vi "VI Server_Get Text Ring Selection.vi"(7 "Label":string, 8 "error in":errorcluster, 9 "Single Instance (T)":bool=TRUE, 11 "VI Server Cluster":T1) -> (0 "error out":errorcluster, 1 "Control Reference":refnum<vi>, 2 "Selection":string, 3 "VI Server Custer.DUP":T1={"Labels"=["Label", "Size", "Font", "Heght", "Width", "Ledding Denominator", "Ledding Nominator", "Label Number", "Microstep Resolution", "X", "Y", "Z", "Italic?", "Underlined?"], "Refs"=[], "VI Ref"=refnum}, 4 "Value":u16, 6 "Label.Text":string)   [LabVIEW 2020, in "VI Server Toolkit LV2013.lvlib"]
doc: "Returns Item Name selected of the Text Ring."
uses:
  VI Server Toolkit LV2013.lvlib
  VI Server_TypeDefs/VI Server_RefsCluster.ctl
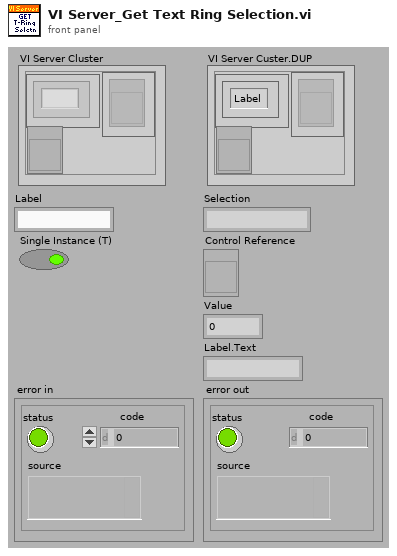
[diagram p1: front panel]
types:
  T1 = typedef "VI Server_RefsCluster.ctl" = cluster{"Labels":string[], "Refs":refnum<vi>[], "VI Ref":refnum<vi>}
  T2 = typedef "LVStringsAndValuesArrayTypeDef_U16.ctl" = cluster{"String":string, "Value":u16}[]
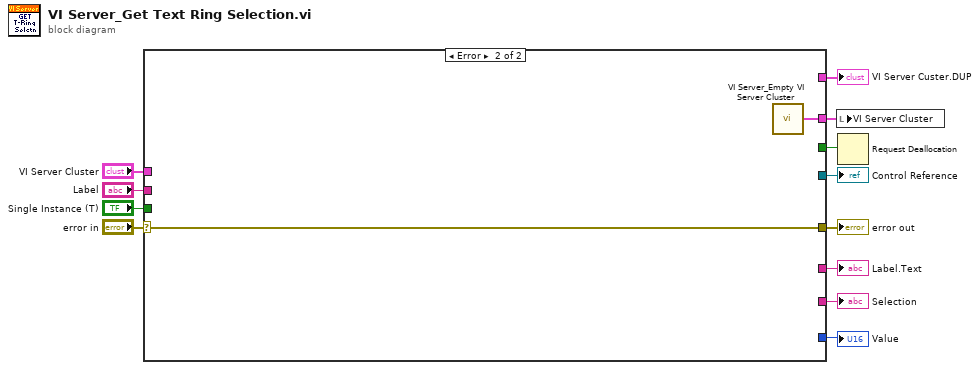
[diagram p0: block diagram]
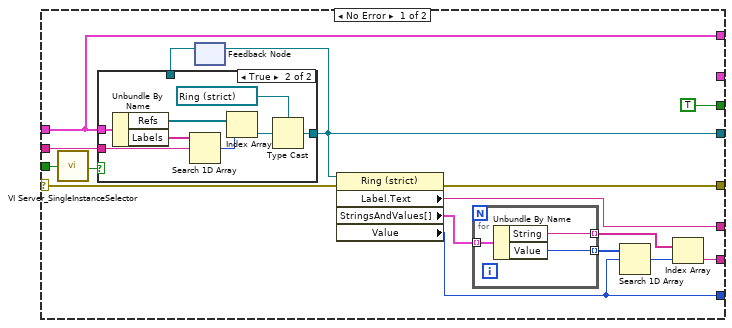
[diagram p2: hidden frame]
diagram:
  n1 = case shown="Error" "error in" {
    selector: "error in" -> [w27 w42]
    tunnel: "Label" -> [w28 _]
    tunnel: "VI Server Cluster" -> [w24 _]
    tunnel: [w26 w42] -> w12
    tunnel: [w14 _] -> w8
    tunnel: [w19 _] -> w7
    tunnel: [w18 _] -> w6
    tunnel: [w25 _] -> w5
    tunnel: [w24 _] -> w4
    tunnel: [TRUE _] -> w3
    tunnel: [_ w41] -> w2
    tunnel: "Single Instance (T)" -> [w15 _]
    frame No Error {
      n2 = call "VI Server_SingleInstanceSelector.vi"("Single Instance (T)"=w15) -> ("Single Instance.OUT"=w16:bool)  [unwired: 6 in]
      n3 = feedback #1() -> (w13:refnum<vi>)  [unwired: 1 in]
      n4 = case shown="True" w16 {
        tunnel: w28 -> [_ w36]
        tunnel: [w29 w31] -> w14
        tunnel: w24 -> [_ w30]
        tunnel: w13 -> [w29 _]
        frame False {
        }
        frame True {
          n5 = Unbundle By Name(w30) -> ("Refs"=w34:refnum<vi>[], "Labels"=w37:string[])
          n6 = Search 1D Array(1D array=w37, element=w36) -> (index of element=w35:i32)  [unwired: 1 out]
          n7 = Index Array(array=w34, index=w35) -> (element=w33:refnum<vi>)
          n8 = Type Cast(type=refnum<vi> refnum ("Ring"), x=w33) -> (*(type *) &x=w31:refnum<vi>)
        }
      }
      n9 = feedback-in #1(w14) -> ()
      n10 = property class="Ring (strict)"(reference=w14, error in=w27) -> (error out=w26:errorcluster, "Label.Text"=w25:string, "StringsAndValues[]"=w23:T2, "Value"=w18:u16)  [unwired: 1 out]
      n11 = for {
        tunnel: w23 -> [w40] mode=indexing
        tunnel: [w39] -> w22 mode=indexing
        tunnel: [w38] -> w20 mode=indexing
        n12 = Unbundle By Name(w40) -> ("String"=w38:string, "Value"=w39:u16)
      }
      n13 = Search 1D Array(1D array=w22, element=w18) -> (index of element=w21:i32)  [unwired: 1 in]
      n14 = Index Array(array=w20, index=w21) -> (element=w19:string)
    }
    frame Error {
      n15 = call "VI Server_Empty VI Server Cluster.vi"() -> ("VI Server Cluster"=w41:T1)  [unwired: 7 in]
    }
  }
  "error out" <- w12
  "VI Server Custer.DUP" <- w4
  "Control Reference" <- w8
  "Selection" <- w7
  "Value" <- w6
  "Label.Text" <- w5
  n16 = local write "VI Server Cluster"(w2) -> ()
  n17 = Request Deallocation(w3) -> ()
